vi "Set Current.vi"(8 "error in (no error)":errorcluster, 10 "Current":dbl, 11 "PS in":refnum<class "PS.lvclass">) -> (0 "error out":errorcluster, 3 "PS out":refnum<class "PS.lvclass">)   [LabVIEW 2020, in "PS.lvlib" / "PS.lvclass"]
uses:
  PS.lvclass
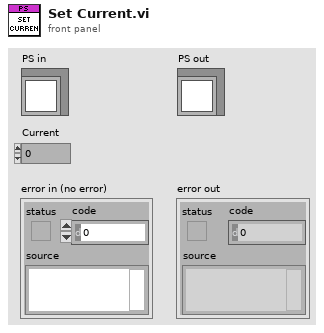
[diagram p1: front panel]
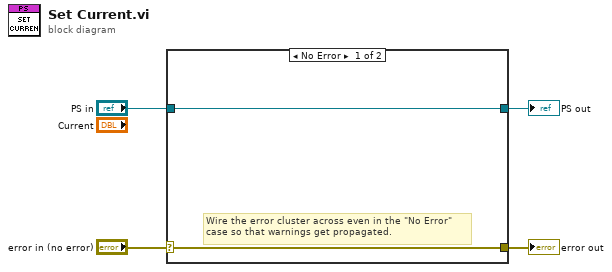
[diagram p0: block diagram]
diagram:
  n1 = case shown="No Error" "error in (no error)" {
    selector: "error in (no error)" -> [w5 w8]
    tunnel: [w5 w8] -> w3
    tunnel: [w6 w7] -> w1
    tunnel: "PS in" -> [w6 w7]
    frame No Error {
      # "Wire the error cluster across even in the \"No Error\"\ncase so that warnings get propagated."
    }
    frame Error {
    }
  }
  "error out" <- w3
  "PS out" <- w1
